vi "Decode TCP Data.vi"(0 "TCP Rx-Tx Cluster In":T8={"Interface"="CPU", "Command"="CPU Info", "SubCmd"="Monitor", "Data"=variant}, 1 "RT-Data's In":T1={"DO Info"={"Channels"=[], "Data"=[], "Time"=""}, "AI-Data From RT--Cluster"={"Channel Name's"=[], "Channel Data's"=[], "Date & Time"=""}, "Hardware Information"=variant(cluster{"Serial Hardware Info JSON Format":cluster{"Command":string, "SubCmd":string, "Channel":string[]}, "Analog HW Info JSON Format":cluster{"Command":string, "SubCmd":string, "Input":string[], "Output":string[]}, "Digital HW Info JSON Format":cluster{"Command":string, "SubCmd":string, "Input":string[], "Output":string[]}, "Ethernet IP Address JSON Format":cluster{"Command":string, "SubCmd":string, "IP":string[]}} {"Serial Hardware Info JSON Format"={"Command"="", "SubCmd"="", "Channel"=[]}, "Analog HW Info JSON Format"={"Command"="", "SubCmd"="", "Input"=[], "Output"=[]}, "Digital HW Info JSON Format"={"Command"="", "SubCmd"="", "Input"=[], "Output"=[]}, "Ethernet IP Address JSON Format"={"Command"="", "SubCmd"="", "IP"=[]}}), "Data Logging Completed?"=FALSE}, 2 "Message Queue out":refnum<class "Delacor_lib_QMH_Message Queue.lvclass">, 11 "error in":errorcluster) -> (3 "RT-Data's Out":T1={"DO Info"={"Channels"=[], "Data"=[], "Time"=""}, "AI-Data From RT--Cluster"={"Channel Name's"=[], "Channel Data's"=[], "Date & Time"=""}, "Hardware Information"=variant(cluster{"Serial Hardware Info JSON Format":cluster{"Command":string, "SubCmd":string, "Channel":string[]}, "Analog HW Info JSON Format":cluster{"Command":string, "SubCmd":string, "Input":string[], "Output":string[]}, "Digital HW Info JSON Format":cluster{"Command":string, "SubCmd":string, "Input":string[], "Output":string[]}, "Ethernet IP Address JSON Format":cluster{"Command":string, "SubCmd":string, "IP":string[]}} {"Serial Hardware Info JSON Format"={"Command"="", "SubCmd"="", "Channel"=[]}, "Analog HW Info JSON Format"={"Command"="", "SubCmd"="", "Input"=[], "Output"=[]}, "Digital HW Info JSON Format"={"Command"="", "SubCmd"="", "Input"=[], "Output"=[]}, "Ethernet IP Address JSON Format"={"Command"="", "SubCmd"="", "IP"=[]}}), "Data Logging Completed?"=FALSE}, 15 "error out":errorcluster)   [LabVIEW 2024]
uses:
  Host-Control's/TCP Tx-Rx cluster.ctl
  Main Engine/Controls/Main Engine Serial Info JSON Data.ctl
  Main Engine/Controls/Main Engine DAQ Harware Info JSON Data.ctl
  Main Engine/Controls/Main Engine Ehernet IP Address JSON Data.ctl
  Host-Control's/RT Data's.ctl
  Host-Control's/DIO Data's from RT.ctl
  Host-Control's/AI-Data from RT.ctl
  <vilib>/Delacor/Delacor QMH/Libraries/Message Queue_class/Delacor_lib_QMH_Message Queue.lvclass
  <vilib>/Delacor/Delacor QMH/Libraries/Message Queue_class/Delacor_lib_QMH_Message Queue.lvclass/Delacor_lib_QMH_Message Queue.ctl
  <vilib>/Delacor/Delacor QMH/Libraries/Message Queue_class/Delacor_lib_QMH_Enqueue Message (Single).vi
panel:
  in  "output cluster":T7
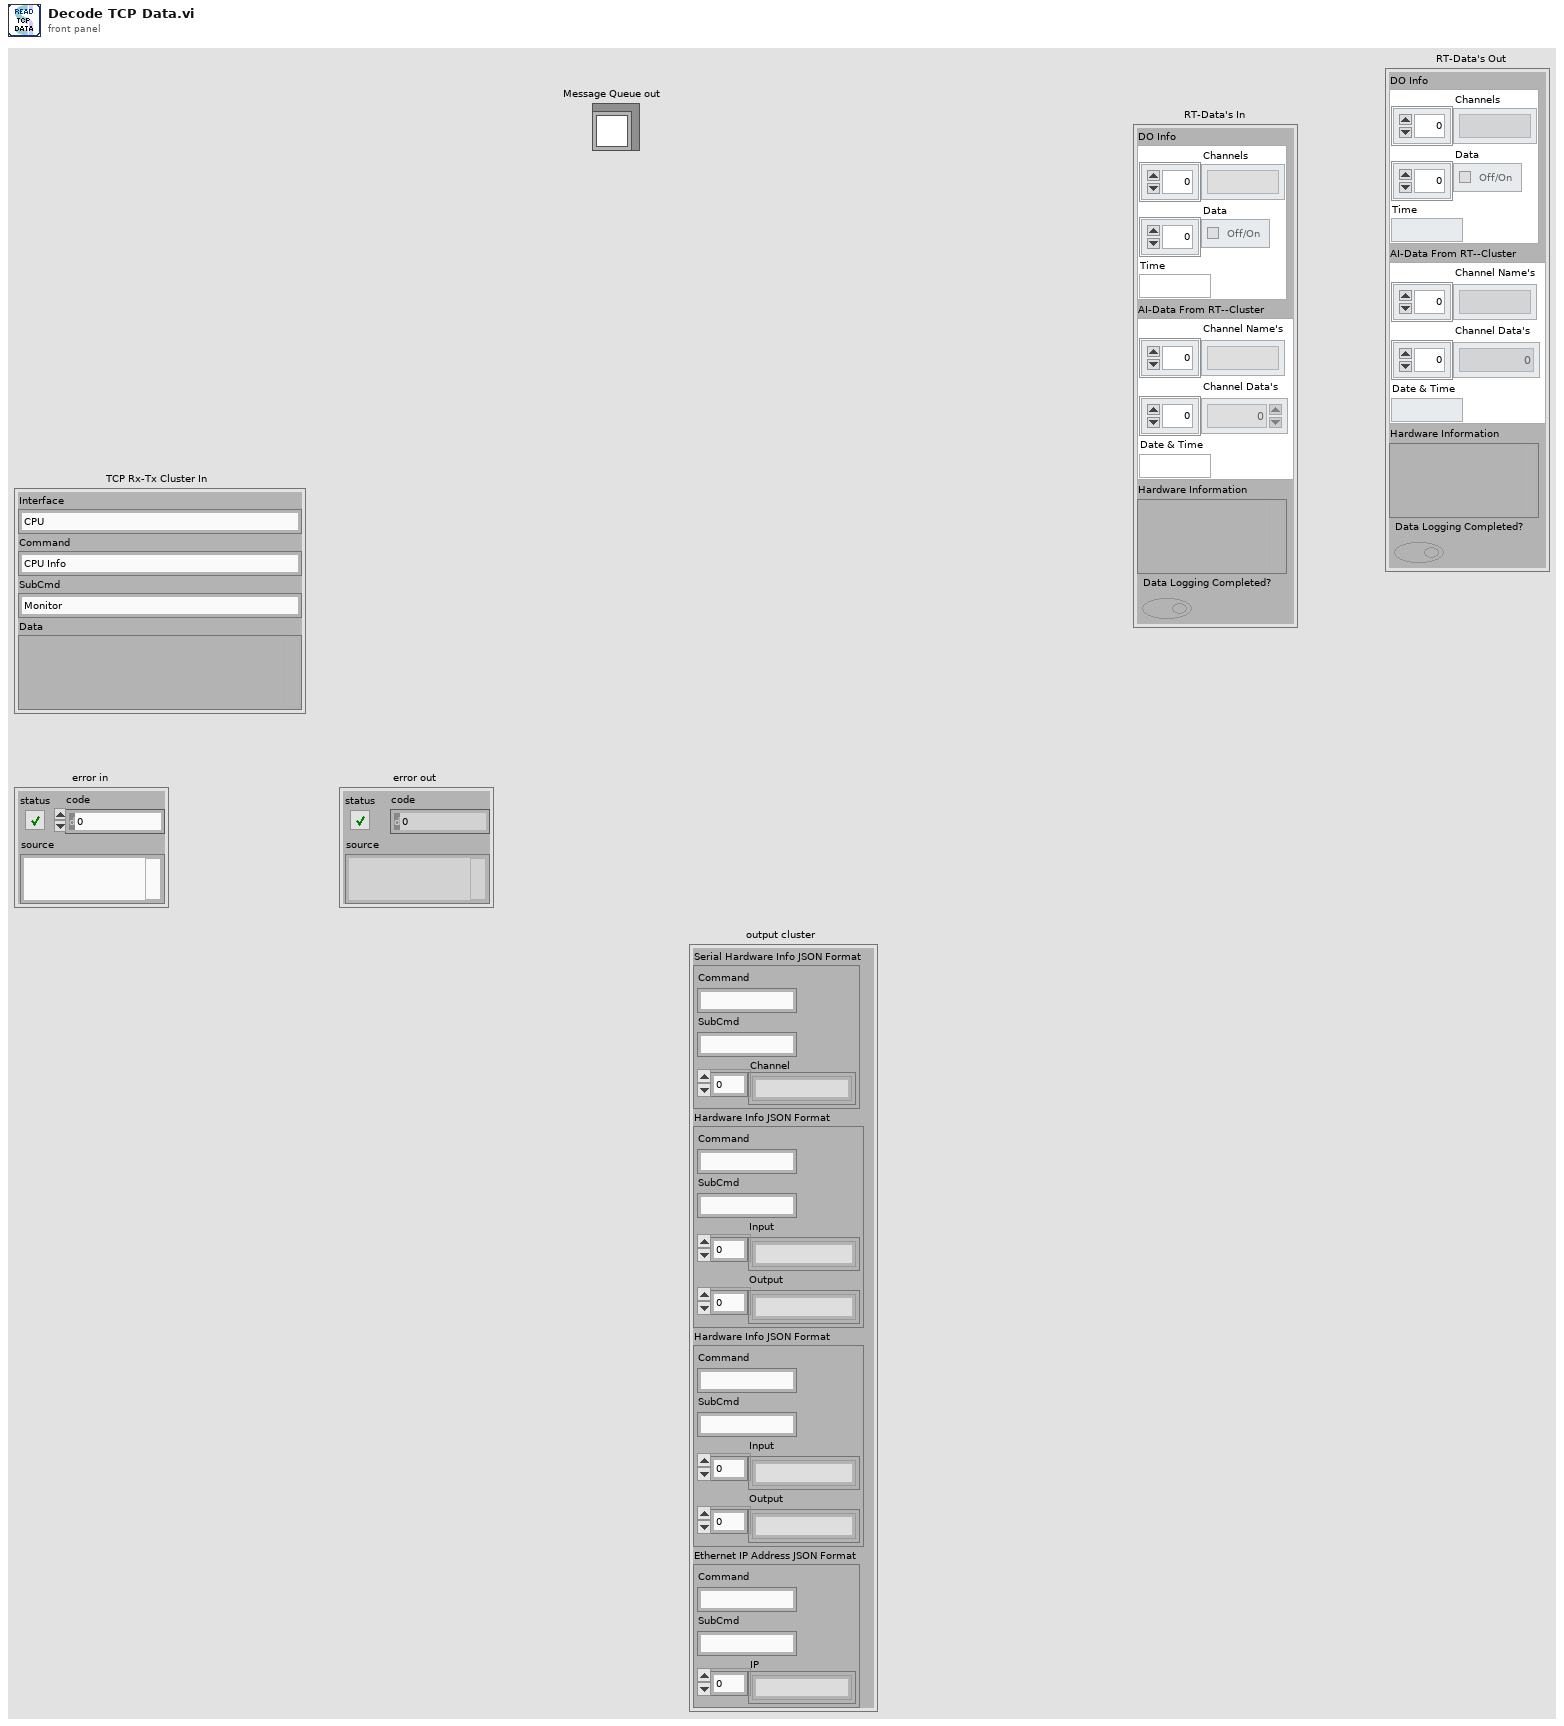
[diagram p1: front panel]
types:
  T1 = typedef "RT Data's.ctl" = cluster{"DO Info":T2, "AI-Data From RT--Cluster":T3, "Hardware Information":variant, "Data Logging Completed?":bool}
  T2 = typedef "DIO Data's from RT.ctl" = cluster{"Channels":string[], "Data":bool[], "Time":string}
  T3 = typedef "AI-Data from RT.ctl" = cluster{"Channel Name's":string[], "Channel Data's":dbl[], "Date & Time":string}
  T4 = typedef "Main Engine Serial Info JSON Data.ctl" = cluster{"Command":string, "SubCmd":string, "Channel":string[]}
  T5 = typedef "Main Engine DAQ Harware Info JSON Data.ctl" = cluster{"Command":string, "SubCmd":string, "Input":string[], "Output":string[]}
  T6 = typedef "Main Engine Ehernet IP Address JSON Data.ctl" = cluster{"Command":string, "SubCmd":string, "IP":string[]}
  T7 = cluster{"Serial Hardware Info JSON Format":T4, "Hardware Info JSON Format":T5, "Hardware Info JSON Format":T5, "Ethernet IP Address JSON Format":T6}
  T8 = typedef "TCP Tx-Rx cluster.ctl" = cluster{"Interface":string, "Command":string, "SubCmd":string, "Data":variant}
  T9 = cluster{"Channels":string[], "Data":i16[], "Time":string}
  T10 = cluster{"Channel":string, "Data":dbl, "Data & Time":string}[]
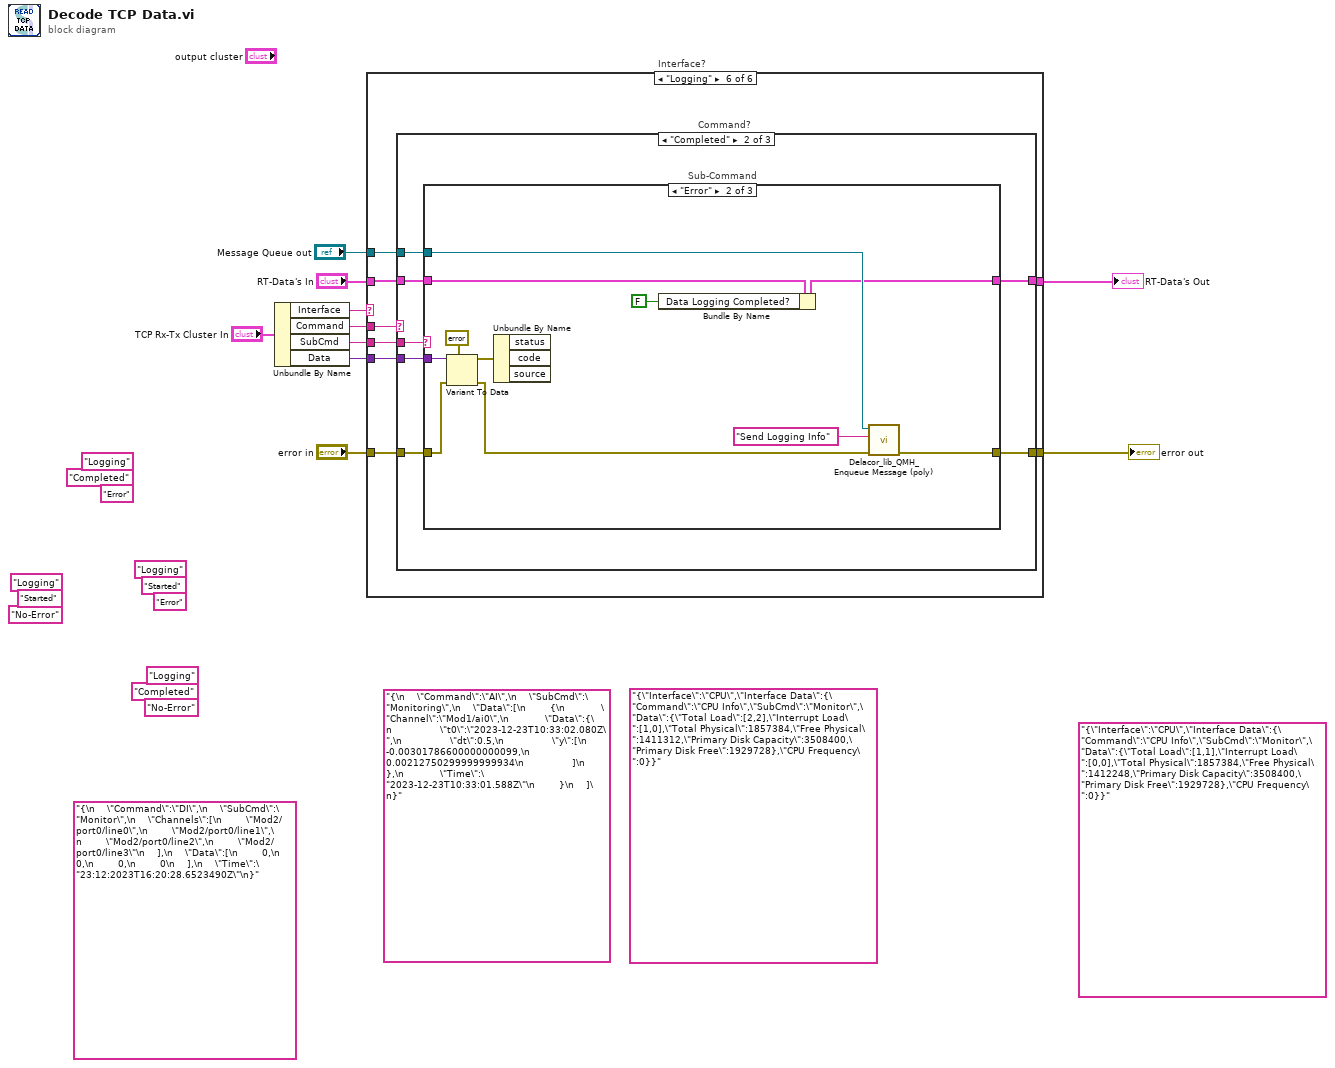
[diagram p0: block diagram]
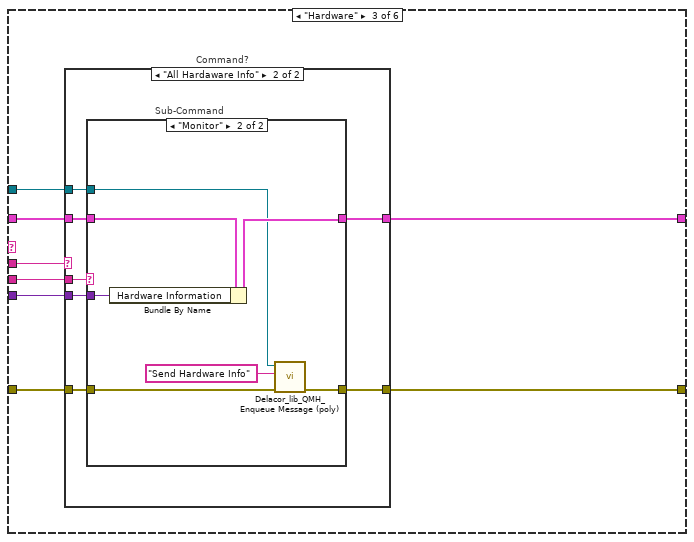
[diagram p6: hidden frame]
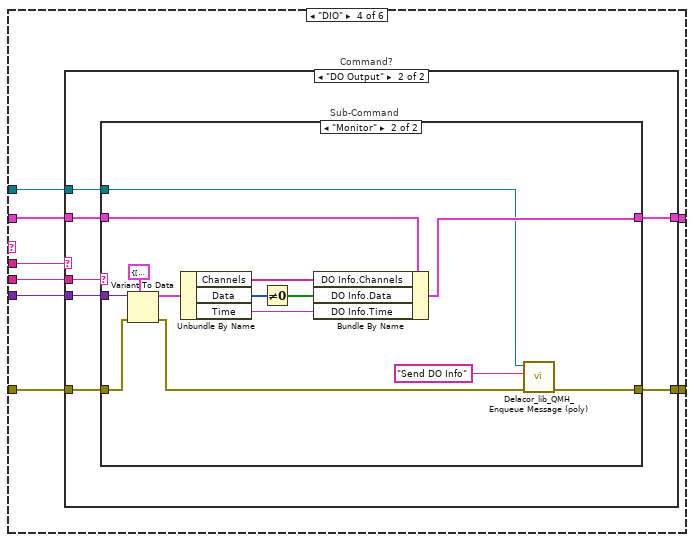
[diagram p9: hidden frame]
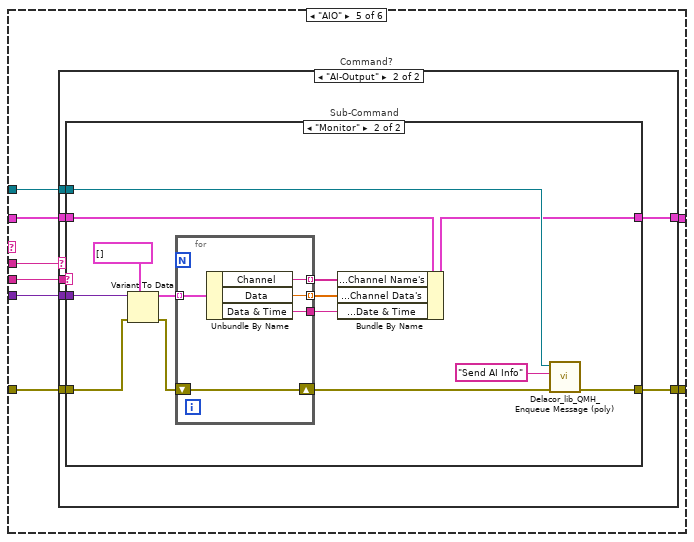
[diagram p12: hidden frame]
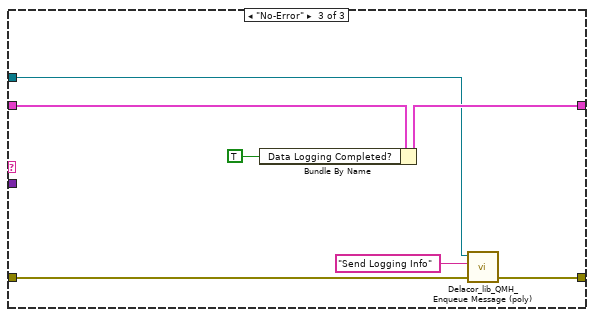
[diagram p17: hidden frame]
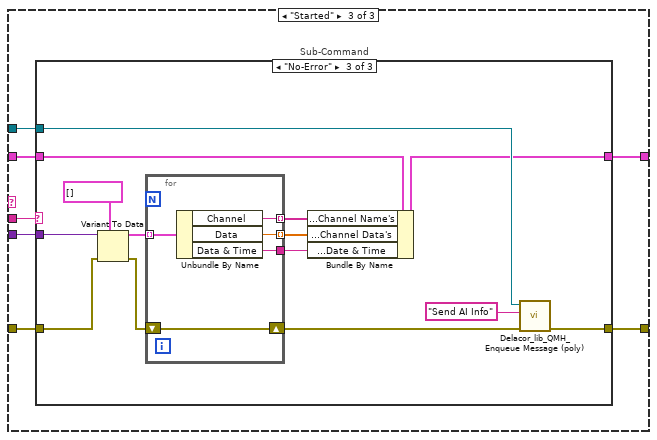
[diagram p18: hidden frame]
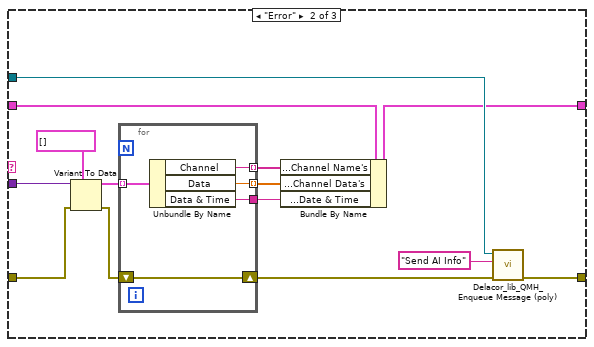
[diagram p20: hidden frame]
diagram:
  (unwired) "Error" ("Interface Data.SubCmd")
  (unwired) "Logging" ("Interface")
  (unwired) "Started" ("Command")
  (unwired) "No-Error" ("Interface Data.SubCmd")
  (unwired) "Logging" ("Interface")
  (unwired) "Started" ("Command")
  (unwired) "No-Error" ("Interface Data.SubCmd")
  (unwired) "Logging" ("Interface")
  (unwired) "Completed" ("Command")
  (unwired) "Error" ("Interface Data.SubCmd")
  (unwired) "Logging" ("Interface")
  (unwired) "Completed" ("Command")
  (unwired) "{\"Interface\":\"CPU\",\"Interface Data\":{\"Command\":\"CPU Info\",\"SubCmd\":\"Monitor\",\"Data\":{\"Total Load\":[1,1],\"Interrupt Load\":[0,0],\"Total Physical\":1857384,\"Free Physical\":1412248,\"Primary Disk Capacity\":3508400,\"Primary Disk Free\":1929728},\"CPU Frequency\":0}}"
  (unwired) "{\"Interface\":\"CPU\",\"Interface Data\":{\"Command\":\"CPU Info\",\"SubCmd\":\"Monitor\",\"Data\":{\"Total Load\":[2,2],\"Interrupt Load\":[1,0],\"Total Physical\":1857384,\"Free Physical\":1411312,\"Primary Disk Capacity\":3508400,\"Primary Disk Free\":1929728},\"CPU Frequency\":0}}"
  (unwired) "{\n    \"Command\":\"AI\",\n    \"SubCmd\":\"Monitoring\",\n    \"Data\":[\n        {\n            \"Channel\":\"Mod1/ai0\",\n            \"Data\":{\n                \"t0\":\"2023-12-23T10:33:02.080Z\",\n                \"dt\":0.5,\n                \"y\":[\n                    -0.00301786600000000099,\n                    0.00212750299999999934\n                ]\n            },\n            \"Time\":\"2023-12-23T10:33:01.588Z\"\n        }\n    ]\n}"
  (unwired) "{\n    \"Command\":\"DI\",\n    \"SubCmd\":\"Monitor\",\n    \"Channels\":[\n        \"Mod2/port0/line0\",\n        \"Mod2/port0/line1\",\n        \"Mod2/port0/line2\",\n        \"Mod2/port0/line3\"\n    ],\n    \"Data\":[\n        0,\n        0,\n        0,\n        0\n    ],\n    \"Time\":\"23:12:2023T16:20:28.6523490Z\"\n}"
  n1 = Unbundle By Name("TCP Rx-Tx Cluster In") -> ("Interface"=w10:string, "Command"=w9:string, "SubCmd"=w8:string, "Data"=w7:variant)
  n2 = case "Interface?" shown="\"Logging\"" w10 {
    tunnel: w9 -> [_ w15 w25 w51 w84 w122]
    tunnel: w8 -> [_ w14 w24 w50 w83 w121]
    tunnel: w7 -> [_ _ w23 w49 w82 w120]
    tunnel: [w12 w16 w21 w47 w80 w118] -> w5
    tunnel: "error in" -> [w12 w16 w22 w48 w81 w119]
    tunnel: [w11 w13 w20 w46 w79 w117] -> w3
    tunnel: "RT-Data's In" -> [w11 w13 w19 w45 w78 w116]
    tunnel: "Message Queue out" -> [_ _ w18 w44 w77 w115]
    frame Default {
    }
    frame "CPU" {
      n3 = case "Command?" shown="\"All Hardaware Info\"" w15 {
        tunnel: w14 -> [_ w17]
        frame Default {
        }
        frame "All Hardaware Info" {
          n4 = case "Sub-Command" shown="\"Monitor\"" w17 {
            frame "False", Default {
            }
            frame "Monitor" {
            }
          }
        }
      }
    }
    frame "Hardware" {
      n5 = case "Command?" shown="\"All Hardaware Info\"" w25 {
        tunnel: w24 -> [_ w34]
        tunnel: w23 -> [_ w33]
        tunnel: w22 -> [w27 w32]
        tunnel: [w27 w31] -> w21
        tunnel: [w26 w30] -> w20
        tunnel: w19 -> [w26 w29]
        tunnel: w18 -> [_ w28]
        frame Default {
        }
        frame "All Hardaware Info" {
          n6 = case "Sub-Command" shown="\"Monitor\"" w34 {
            tunnel: w33 -> [_ w38]
            tunnel: w32 -> [w36 w37]
            tunnel: [w36 w39] -> w31
            tunnel: [w35 w42] -> w30
            tunnel: w29 -> [w35 w43]
            tunnel: w28 -> [_ w41]
            frame Default {
            }
            frame "Monitor" {
              n7 = Bundle By Name(cluster=w43, "Hardware Information"=w38) -> (w42:T1)
              n8 = call-poly <vilib>:"Delacor_lib_QMH_Enqueue Message (poly).vi"("error in"=w37, "Message"="Send Hardware Info", "Message Queue in"=w41) -> ("error out"=w39:errorcluster)  [unwired: 7 in, 1 out]
            }
          }
        }
      }
    }
    frame "DIO" {
      n9 = case "Command?" shown="\"DO Output\"" w51 {
        tunnel: w50 -> [_ w60]
        tunnel: w49 -> [_ w59]
        tunnel: w48 -> [w53 w58]
        tunnel: [w53 w57] -> w47
        tunnel: [w52 w56] -> w46
        tunnel: w45 -> [w52 w55]
        tunnel: w44 -> [_ w54]
        frame Default {
        }
        frame "DO Output" {
          n10 = case "Sub-Command" shown="\"Monitor\"" w60 {
            tunnel: w59 -> [_ w76]
            tunnel: w58 -> [w62 w75]
            tunnel: [w62 w63] -> w57
            tunnel: [w61 w70] -> w56
            tunnel: w55 -> [w61 w71]
            tunnel: w54 -> [_ w65]
            frame Default {
            }
            frame "Monitor" {
              n11 = Variant To Data(error in=w75, type=T9 {"Channels"=[], "Data"=[], "Time"=""} ("cluster"), Variant=w76) -> (data=w73:T9, error out=w64:errorcluster)
              n12 = Unbundle By Name(w73) -> ("Channels"=w69:string[], "Data"=w72:i16[], "Time"=w68:string)
              n13 = Not Equal To 0?(x=w72) -> (x != 0?=w67:bool[])
              n14 = Bundle By Name(cluster=w71, "DO Info.Channels"=w69, "DO Info.Data"=w67, "DO Info.Time"=w68) -> (w70:T1)
              n15 = call-poly <vilib>:"Delacor_lib_QMH_Enqueue Message (poly).vi"("error in"=w64, "Message"="Send DO Info", "Message Queue in"=w65) -> ("error out"=w63:errorcluster)  [unwired: 7 in, 1 out]
            }
          }
        }
      }
    }
    frame "AIO" {
      n16 = case "Command?" shown="\"AI-Output\"" w84 {
        tunnel: w83 -> [_ w93]
        tunnel: w82 -> [_ w92]
        tunnel: w81 -> [w86 w91]
        tunnel: [w86 w90] -> w80
        tunnel: [w85 w89] -> w79
        tunnel: w78 -> [w85 w88]
        tunnel: w77 -> [_ w87]
        frame Default {
        }
        frame "AI-Output" {
          n17 = case "Sub-Command" shown="\"Monitor\"" w93 {
            tunnel: w92 -> [_ w109]
            tunnel: w91 -> [w95 w108]
            tunnel: [w95 w96] -> w90
            tunnel: [w94 w102] -> w89
            tunnel: w88 -> [w94 w103]
            tunnel: w87 -> [_ w106]
            frame Default {
            }
            frame "Monitor" {
              n18 = Variant To Data(error in=w108, type=T10 [] ("AI-Data Out"), Variant=w109) -> (data=w105:T10, error out=w98:errorcluster)
              n19 = for {
                tunnel: w105 -> [w114] mode=indexing
                tunnel: [w113] -> w101 mode=indexing
                tunnel: [w112] -> w99
                tunnel: [w111] -> w100 mode=indexing
                shift-right: [w110] -> w97
                shift-left: w98 -> [w110]
                n20 = Unbundle By Name(w114) -> ("Channel"=w113:string, "Data"=w111:dbl, "Data & Time"=w112:string)
              }
              n21 = Bundle By Name(cluster=w103, "AI-Data From RT--Cluster.Channel Name's"=w101, "AI-Data From RT--Cluster.Channel Data's"=w100, "AI-Data From RT--Cluster.Date & Time"=w99) -> (w102:T1)
              n22 = call-poly <vilib>:"Delacor_lib_QMH_Enqueue Message (poly).vi"("error in"=w97, "Message"="Send AI Info", "Message Queue in"=w106) -> ("error out"=w96:errorcluster)  [unwired: 7 in, 1 out]
            }
          }
        }
      }
    }
    frame "Logging" {
      n23 = case "Command?" shown="\"Completed\"" w122 {
        tunnel: w121 -> [_ w131 w157]
        tunnel: w120 -> [_ w130 w156]
        tunnel: w119 -> [w124 w129 w155]
        tunnel: [w124 w128 w154] -> w118
        tunnel: [w123 w127 w153] -> w117
        tunnel: w116 -> [w123 w126 w152]
        tunnel: w115 -> [_ w125 w151]
        frame Default {
        }
        frame "Completed" {
          n24 = case "Sub-Command" shown="\"Error\"" w131 {
            tunnel: w130 -> [_ w144 _]
            tunnel: w129 -> [w133 w143 w150]
            tunnel: [w133 w139 w150] -> w128
            tunnel: [w132 w135 w148] -> w127
            tunnel: w126 -> [w132 w136 w149]
            tunnel: w125 -> [_ w138 w145]
            frame Default {
            }
            frame "Error" {
              n25 = Variant To Data(error in=w143, type=errorcluster {"status"=FALSE, "code"=0, "source"=""} ("error constant"), Variant=w144) -> (data=w142:errorcluster, error out=w140:errorcluster)
              n26 = Unbundle By Name(w142) -> ()  [unwired: 3 out]
              n27 = Bundle By Name(cluster=w136, "Data Logging Completed?"=FALSE) -> (w135:T1)
              n28 = call-poly <vilib>:"Delacor_lib_QMH_Enqueue Message (poly).vi"("error in"=w140, "Message"="Send Logging Info", "Message Queue in"=w138) -> ("error out"=w139:errorcluster)  [unwired: 7 in, 1 out]
            }
            frame "No-Error" {
              n29 = Bundle By Name(cluster=w149, "Data Logging Completed?"=TRUE) -> (w148:T1)
              n30 = call-poly <vilib>:"Delacor_lib_QMH_Enqueue Message (poly).vi"("Message"="Send Logging Info", "Message Queue in"=w145) -> ()  [unwired: 8 in, 2 out]
            }
          }
        }
        frame "Started" {
          n31 = case "Sub-Command" shown="\"No-Error\"" w157 {
            tunnel: w156 -> [_ w173 w192]
            tunnel: w155 -> [w159 w172 w191]
            tunnel: [w159 w160 w179] -> w154
            tunnel: [w158 w166 w185] -> w153
            tunnel: w152 -> [w158 w167 w186]
            tunnel: w151 -> [_ w170 w189]
            frame Default {
            }
            frame "Error" {
              n32 = Variant To Data(error in=w172, type=T10 [] ("AI-Data Out"), Variant=w173) -> (data=w169:T10, error out=w162:errorcluster)
              n33 = for {
                tunnel: w169 -> [w178] mode=indexing
                tunnel: [w177] -> w165 mode=indexing
                tunnel: [w176] -> w163
                tunnel: [w175] -> w164 mode=indexing
                shift-right: [w174] -> w161
                shift-left: w162 -> [w174]
                n34 = Unbundle By Name(w178) -> ("Channel"=w177:string, "Data"=w175:dbl, "Data & Time"=w176:string)
              }
              n35 = Bundle By Name(cluster=w167, "AI-Data From RT--Cluster.Channel Name's"=w165, "AI-Data From RT--Cluster.Channel Data's"=w164, "AI-Data From RT--Cluster.Date & Time"=w163) -> (w166:T1)
              n36 = call-poly <vilib>:"Delacor_lib_QMH_Enqueue Message (poly).vi"("error in"=w161, "Message"="Send AI Info", "Message Queue in"=w170) -> ("error out"=w160:errorcluster)  [unwired: 7 in, 1 out]
            }
            frame "No-Error" {
              n37 = Variant To Data(error in=w191, type=T10 [] ("AI-Data Out"), Variant=w192) -> (data=w188:T10, error out=w181:errorcluster)
              n38 = for {
                tunnel: w188 -> [w197] mode=indexing
                tunnel: [w196] -> w184 mode=indexing
                tunnel: [w195] -> w182
                tunnel: [w194] -> w183 mode=indexing
                shift-right: [w193] -> w180
                shift-left: w181 -> [w193]
                n39 = Unbundle By Name(w197) -> ("Channel"=w196:string, "Data"=w194:dbl, "Data & Time"=w195:string)
              }
              n40 = Bundle By Name(cluster=w186, "AI-Data From RT--Cluster.Channel Name's"=w184, "AI-Data From RT--Cluster.Channel Data's"=w183, "AI-Data From RT--Cluster.Date & Time"=w182) -> (w185:T1)
              n41 = call-poly <vilib>:"Delacor_lib_QMH_Enqueue Message (poly).vi"("error in"=w180, "Message"="Send AI Info", "Message Queue in"=w189) -> ("error out"=w179:errorcluster)  [unwired: 7 in, 1 out]
            }
          }
        }
      }
    }
  }
  "error out" <- w5
  "RT-Data's Out" <- w3
